vi "ButtonsGlobal.vi"(8 "Action":enum16{"Set", "Get"}(ring), 11 "Input":T2) -> (3 "Output":T2)   [LabVIEW 2021]
uses:
  <vilib>/sound2/lvsound2.llb/Sound File Refnum.ctl
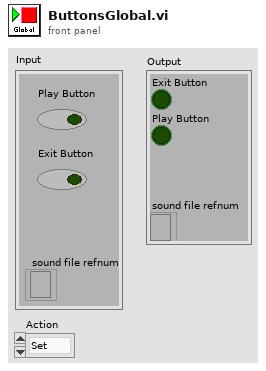
[diagram p1: front panel]
types:
  T1 = typedef "Sound File Refnum.ctl" = refnum<file>
  T2 = cluster{"Exit Button":bool, "Play Button":bool, "sound file refnum":T1}
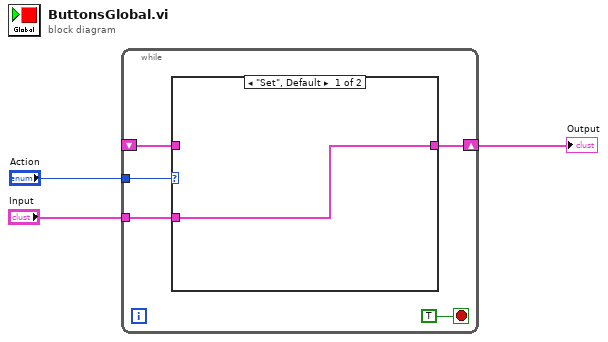
[diagram p0: block diagram]
diagram:
  n1 = while {
    tunnel: "Input" -> [w7]
    tunnel: "Action" -> [w8]
    shift-right: [w6] -> w2
    shift-left: _ -> [w5]
    stop <- TRUE stop-if-true
    n2 = case shown="\"Set\", Default" w8 {
      tunnel: w7 -> [w9 _]
      tunnel: [w9 w10] -> w6
      tunnel: w5 -> [_ w10]
      frame "Set", Default {
      }
      frame "Get" {
      }
    }
  }
  "Output" <- w2
